vi "CorrelationTest3.vi"() -> ()   [LabVIEW 2014]
uses:
  <userlib>/Nanonis Prog Interface V5/Nanonis Prog Interface.lvlib
panel:
  out "element":i32
  in  "length":i32
  in  "method":i32 min=0 max=20
  out "Pixelated 2":picture
  out "Y drift 2":i32
  out "X drift 2":i32
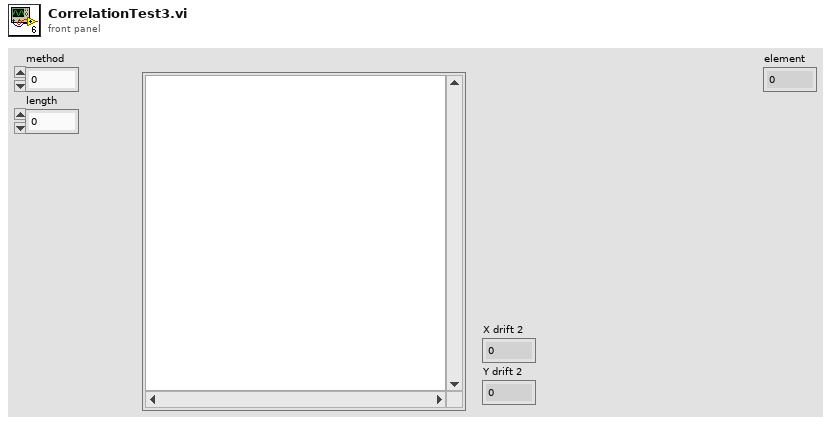
[diagram p1: front panel]
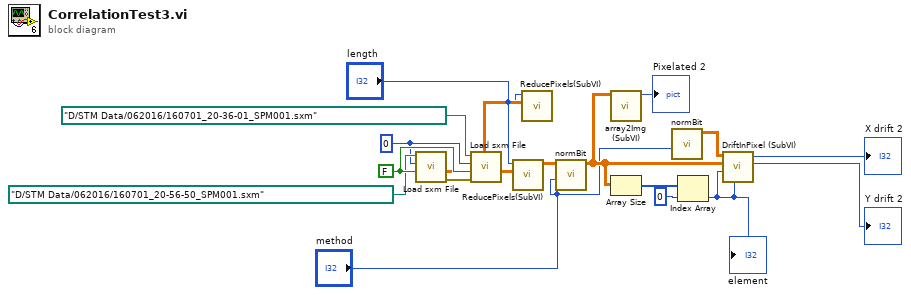
[diagram p0: block diagram]
diagram:
  w4 = i8 0 ("Read channel")
  w18 = FALSE ("Scan direction")
  n1 = call <userlib>:"Load sxm File.vi"("Scan direction"=w18, "Read channel"=w4, "Scan data file"=path "D:/STM Data/062016/160701_20-56-50_SPM001.sxm") -> ("error out"=w17:errorcluster, "Data"=w2:sgl[][])  [unwired: 3 in, 4 out]
  n2 = call <userlib>:"Load sxm File.vi"("error in"=w17, "Scan direction"=w18, "Read channel"=w4, "Scan data file"=path "D:/STM Data/062016/160701_20-36-01_SPM001.sxm") -> ("Data"=w14:sgl[][])  [unwired: 2 in, 5 out]
  n3 = call "ReducePixels(SubVI).vi"("Array in"=w14, "length"="length") -> ("Array out"=w13:dbl[][])  [unwired: 9 in]
  n4 = call "ReducePixels(SubVI).vi"("Array in"=w2, "length"="length") -> ()  [unwired: 9 in, 1 out]
  n5 = call "normBit.vi"("method"="method", "Rxy"=w13) -> ("Array"=w5:dbl[][])  [unwired: 8 in, 1 out]
  n6 = call "array2Img (SubVI).vi"("Rxy"=w5) -> ("new picture"=→"Pixelated 2":picture)  [unwired: 10 in]
  n7 = Array Size(array=w5) -> (size(s)=w9:i32[])
  n8 = call "normBit.vi"("method"="method") -> ("Array"=w12:dbl[][])  [unwired: 9 in, 1 out]
  n9 = Index Array(array=w9, index=0) -> (element=w8:i32)
  "element" <- w8
  n10 = call "DriftInPixel (SubVI).vi"(6:w8, 9:w8, "New image"=w5, "Ref image"=w12) -> ("Y drift"=→"Y drift 2":i32, "X drift"=→"X drift 2":i32)  [unwired: 5 in, 1 out]
